vi "Row_Sum and Cumulative_Col_Sum.vi"(0 "Image_2d":i16[][](array[numeric]), 5 "error in (no error)":errorcluster) -> (14 "Row_Sum":i16[](array[numeric]), 15 "Col_Sum":i16[](array[numeric]), 16 "Cum_Col_Sum":i16[](array[numeric]), 19 "error out":errorcluster)   [LabVIEW 2015]
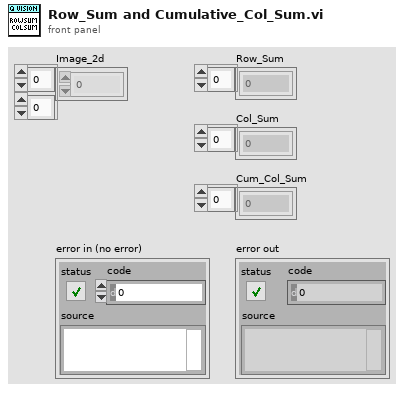
[diagram p1: front panel]
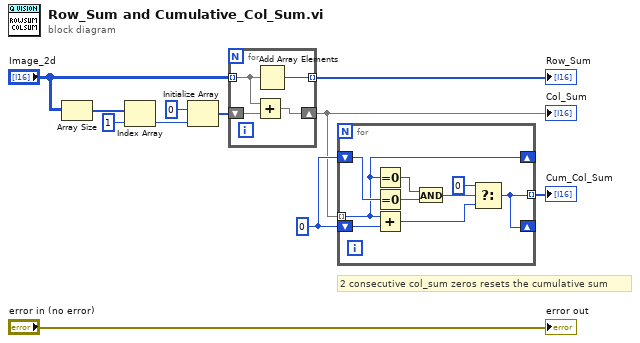
[diagram p0: block diagram]
diagram:
  w3 = i16 0
  # "2 consecutive col_sum zeros resets the cumulative sum"
  n1 = Array Size(array="Image_2d") -> (size(s)=w7:i32[])
  n2 = Index Array(array=w7, index=1) -> (element=w9:i32)
  n3 = Initialize Array(i16 0 ("element"), w9) -> (w8:i16[])
  n4 = for {
    tunnel: "Image_2d" -> [w14] mode=indexing
    shift-right: [w13] -> w1
    shift-left: w8 -> [w15]
    tunnel: [w12] -> w11 mode=indexing
    n5 = Add(x=w14, y=w15) -> (x+y=w13:i16[])
    n6 = Add Array Elements(numeric array=w14) -> (sum=w12:i16)
  }
  "Row_Sum" <- w11
  "Col_Sum" <- w1
  n7 = for {
    tunnel: w1 -> [w21] mode=indexing
    shift-right: [w21] -> _
    shift-left: w3 -> [w24]
    shift-right: [w16] -> _
    shift-left: w3 -> [w20]
    tunnel: [w16] -> w2 mode=indexing
    n8 = Equal To 0?(x=w21) -> (x = 0?=w23:bool)
    n9 = Equal To 0?(x=w24) -> (x = 0?=w22:bool)
    n10 = Add(x=w21, y=w20) -> (x+y=w18:i16)
    n11 = And(x=w23, y=w22) -> (x .and. y?=w19:bool)
    n12 = Select(t=i16 0, s=w19, f=w18) -> (s? t:f=w16:i16)
  }
  "Cum_Col_Sum" <- w2
  "error out" <- "error in (no error)"
